vi "FEA_Model_Unpinned_BC.vi"(11 "FEA_Model in":refnum<class "FEA_Model.lvclass">) -> (3 "FEA_Model out":refnum<class "FEA_Model.lvclass">)   [LabVIEW 2021, in "FEA_Model.lvclass"]
uses:
  FEA_Model.lvclass
  FEA_Model.lvclass/FEA_Model.ctl
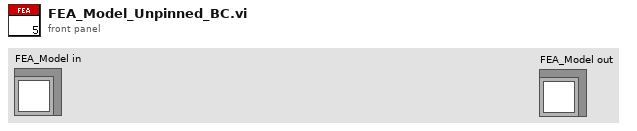
[diagram p1: front panel]
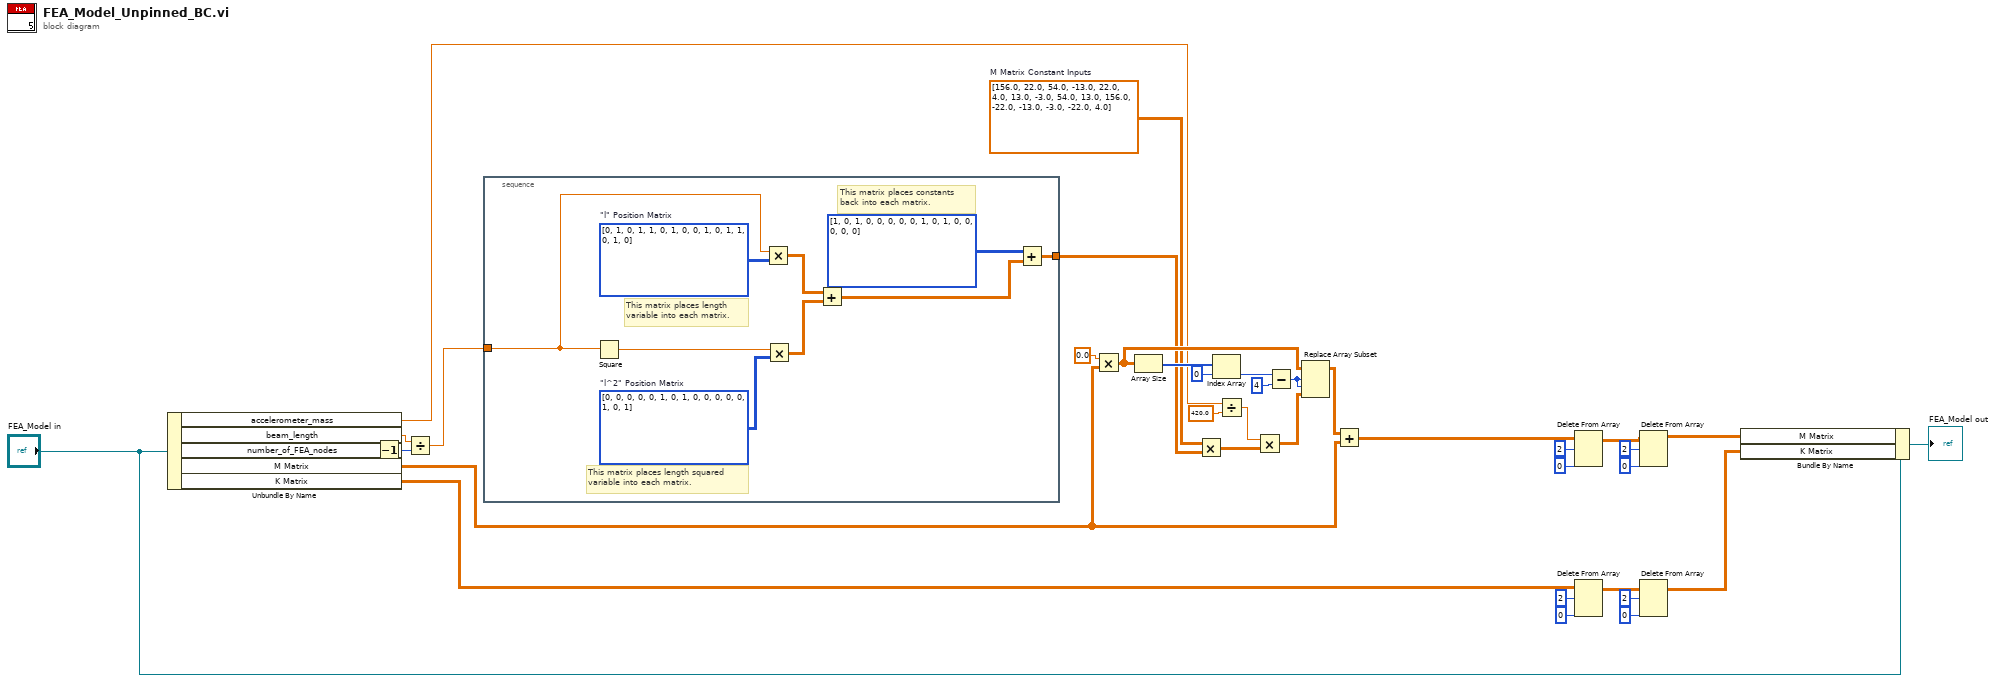
[diagram p0: block diagram]
diagram:
  w26 = dbl[][] [[156.0, 22.0, 54.0, -13.0], [22.0, 4.0, 13.0, -3.0], [54.0, 13.0, 156.0, -22.0], [-13.0, -3.0, -22.0, 4.0]]  # M Matrix Constant Inputs
  n1 = Unbundle By Name("FEA_Model in") -> ("accelerometer_mass"=w17:dbl, "beam_length"=w14:dbl, "number_of_FEA_nodes"=w16:i32, "M Matrix"=w12:dbl[][], "K Matrix"=w11:dbl[][])
  n2 = Decrement(x=w16) -> (x-1=w15:i32)
  n3 = Divide(x=w14, y=w15) -> (x/y=w13:dbl)
  n4 = stacked-sequence {
    tunnel: [w43] -> w28
    tunnel: w13 -> [w45]
    frame #0 {
      w38 = i32[][] [[0, 0, 0, 0], [0, 1, 0, 1], [0, 0, 0, 0], [0, 1, 0, 1]]  # "l^2" Position Matrix
      w37 = i32[][] [[0, 1, 0, 1], [1, 0, 1, 0], [0, 1, 0, 1], [1, 0, 1, 0]]  # "l" Position Matrix
      # "This matrix places length squared\nvariable into each matrix."
      # "This matrix places length \nvariable into each matrix."
      # "This matrix places constants\nback into each matrix."
      n5 = Square(x=w45) -> (x^2=w40:dbl)
      n6 = Multiply(x=w45, y=w37) -> (x*y=w39:dbl[][])
      n7 = Multiply(x=w40, y=w38) -> (x*y=w41:dbl[][])
      n8 = Add(x=w39, y=w41) -> (x+y=w44:dbl[][])
      n9 = Add(x=i32[][] [[1, 0, 1, 0], [0, 0, 0, 0], [1, 0, 1, 0], [0, 0, 0, 0]], y=w44) -> (x+y=w43:dbl[][])
    }
  }
  n10 = Multiply(x=0.0, y=w12) -> (x*y=w29:dbl[][])
  n11 = Array Size(array=w29) -> (size(s)=w30:i32[])
  n12 = Multiply(x=w26, y=w28) -> (x*y=w25:dbl[][])
  n13 = Index Array(array=w30, index=0) -> (element=w32:i32)
  n14 = Divide(x=w17, y=420.0) -> (x/y=w24:dbl)
  n15 = Multiply(x=w24, y=w25) -> (x*y=w35:dbl[][])
  n16 = Subtract(x=w32, y=4) -> (x-y=w34:i32)
  n17 = Replace Array Subset(array=w29, new element=w35, index (row)=w34, index (col)=w34) -> (w36:dbl[][])
  n18 = Add(x=w36, y=w12) -> (x+y=w5:dbl[][])
  n19 = Delete From Array(array=w5, length=2, index (col)=0 ("disabled index (col)")) -> (array with subset deleted=w6:dbl[][])  [unwired: 1 in, 1 out]
  n20 = Delete From Array(array=w11, length=2, index (col)=0 ("disabled index (col)")) -> (array with subset deleted=w18:dbl[][])  [unwired: 1 in, 1 out]
  n21 = Delete From Array(array=w6, length=2, index (row)=0 ("disabled index (col)")) -> (array with subset deleted=w4:dbl[][])  [unwired: 1 in, 1 out]
  n22 = Delete From Array(array=w18, length=2, index (row)=0 ("disabled index (col)")) -> (array with subset deleted=w3:dbl[][])  [unwired: 1 in, 1 out]
  n23 = Bundle By Name(cluster="FEA_Model in", "M Matrix"=w4, "K Matrix"=w3) -> (→"FEA_Model out":refnum<class "FEA_Model.lvclass">)
